vi "stim config array to bool odor matrix (subVI).vi"(9 "num solenoids (10)":i32=10, 10 "stim. config []":T1 {"right odor"."port-odor ring" items=["off"]; "middle odor"."port-odor ring" items=["off"]; "left odor"."port-odor ring" items=["off"]}) -> (1 "string stim. matrix":string[][](array[string]), 2 "bool stim. matrix":bool[][](array[boolean]), 4 "duration []":dbl[](array[numeric]))   [LabVIEW 2021]
uses:
  type-defs/stimulation configuration array (type def).ctl
  type-defs/stimulator configuration line cluster (type def).ctl
  type-defs/port-odor with color cluster (type def).ctl
  type-defs/port-odor ring (type def).ctl
  type-defs/odor color (type def).ctl
  global-variables/global variables.vi
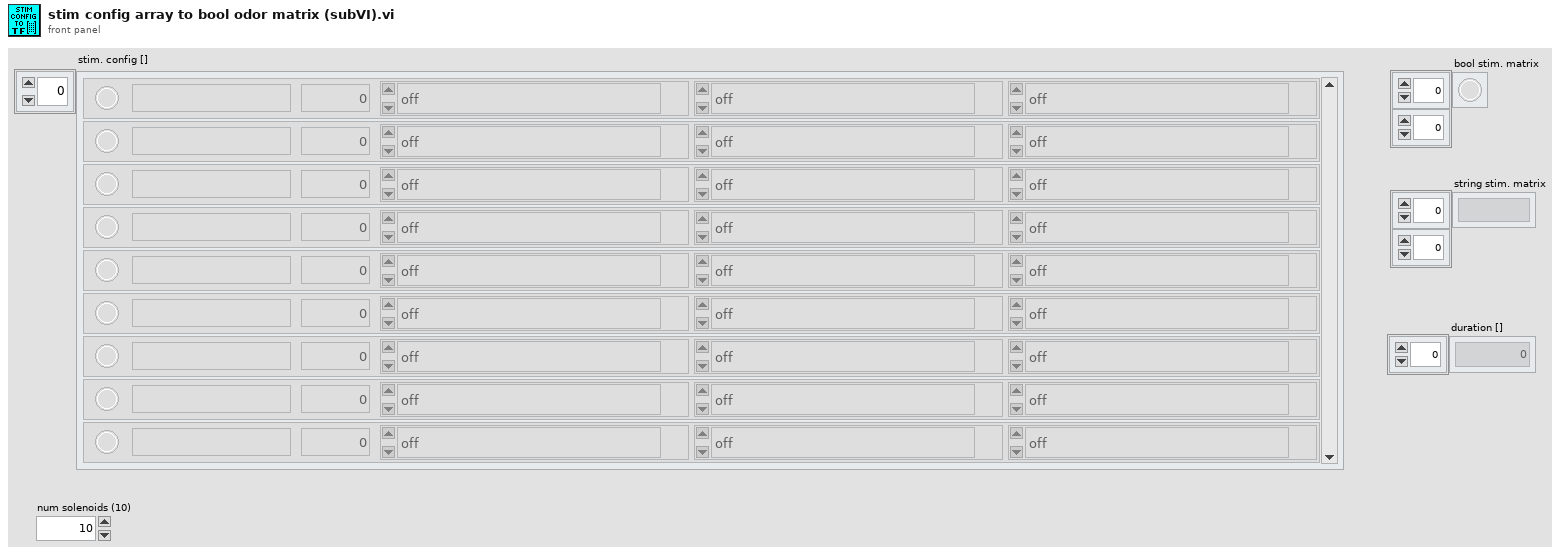
[diagram p1: front panel]
types:
  T1 = typedef "stimulation configuration array (type def).ctl" = T2[]
  T2 = typedef "stimulator configuration line cluster (type def).ctl" = cluster{"description":string, "duration, s":dbl, "left odor":T3, "middle odor":T3, "right odor":T3, "selected?":bool}
  T3 = typedef "port-odor with color cluster (type def).ctl" = cluster{"port-odor ring":T4, "odor color":T5}
  T4 = typedef "port-odor ring (type def).ctl" = u16
  T5 = typedef "odor color (type def).ctl" = u16
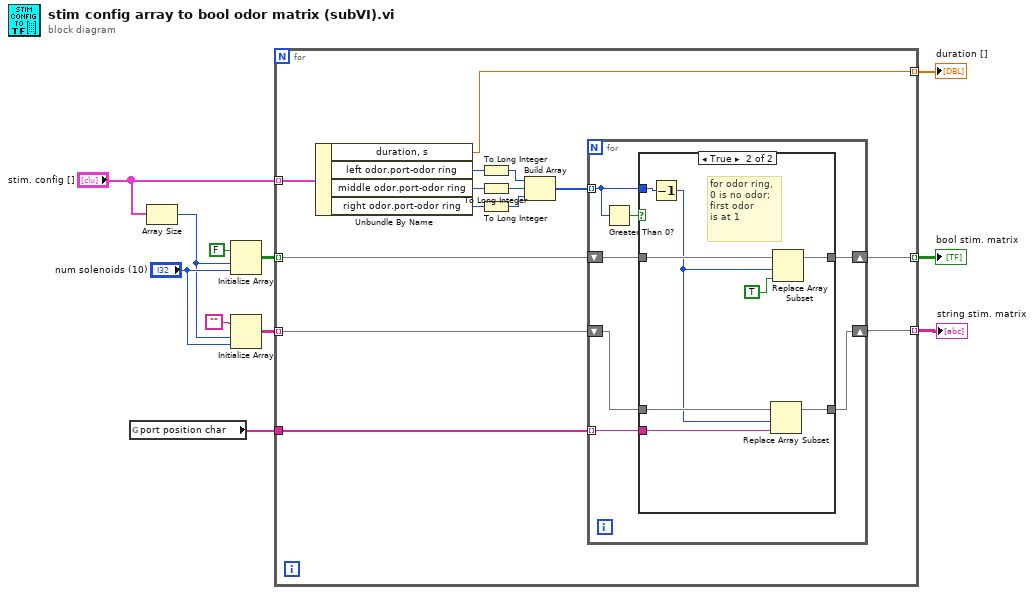
[diagram p0: block diagram]
diagram:
  n1 = global read "global variables.vi" "port position char"() -> (w2:string[])
  n2 = Array Size(array="stim. config []") -> (size(s)=w4:i32)
  n3 = Initialize Array(FALSE, w4, "num solenoids (10)") -> (w9:bool[][])
  n4 = Initialize Array("", w4, "num solenoids (10)") -> (w3:string[][])
  n5 = for {
    tunnel: "stim. config []" -> [w25] mode=indexing
    tunnel: [w24] -> w7 mode=indexing
    tunnel: w9 -> [w16] mode=indexing
    tunnel: [w15] -> w8 mode=indexing
    tunnel: w3 -> [w14] mode=indexing
    tunnel: w2 -> [w13]
    tunnel: [w12] -> w1 mode=indexing
    n6 = Unbundle By Name(w25) -> ("duration, s"=w24:dbl, "left odor.port-odor ring"=w23:T4, "middle odor.port-odor ring"=w22:T4, "right odor.port-odor ring"=w21:T4)
    n7 = To Long Integer(number=w23) -> (32bit integer=w20:i32)
    n8 = To Long Integer(number=w22) -> (32bit integer=w19:i32)
    n9 = To Long Integer(number=w21) -> (32bit integer=w18:i32)
    n10 = Build Array(w20, w19, w18) -> (w17:i32[])
    n11 = for {
      tunnel: w17 -> [w31] mode=indexing
      shift-right: [w29] -> w15
      shift-left: w16 -> [w30]
      shift-right: [w26] -> w12
      shift-left: w14 -> [w28]
      tunnel: w13 -> [w27] mode=indexing
      n12 = Greater Than 0?(x=w31) -> (x > 0?=w32:bool)
      n13 = case shown="True" w32 {
        tunnel: w31 -> [_ w39]
        tunnel: w30 -> [w34 w42]
        tunnel: [w34 w40] -> w29
        tunnel: w28 -> [w33 w38]
        tunnel: w27 -> [_ w37]
        tunnel: [w33 w36] -> w26
        frame False {
        }
        frame True {
          # "for odor ring, \n0 is no odor;\nfirst odor \nis at 1"
          n14 = Decrement(x=w39) -> (x-1=w35:i32)
          n15 = Replace Array Subset(array=w38, new element=w37, index=w35) -> (w36:string[])
          n16 = Replace Array Subset(array=w42, new element=TRUE ("new element/subarray"), index=w35) -> (w40:bool[])
        }
      }
    }
  }
  "bool stim. matrix" <- w8
  "duration []" <- w7
  "string stim. matrix" <- w1
